vi "Disconnect SMU Resources from site.vi"(0 "TSM context":T1, 5 "Site Relays(T)/Non-Site(F)?":bool, 11 "error in":errorcluster) -> (4 "TSM context out":T1, 15 "error out":errorcluster)   [LabVIEW 2019]
doc: "This VI is used to disconnect SMU resources safely by preventing potetial OCP errors."
uses:
  <vilib>/NI_TestStand_SemiconductorModule/NI_TestStand_Semiconductor_Module.lvlibp/PinMap/General/SemiconductorModuleContext.ctl
  <vilib>/NI_TestStand_SemiconductorModule/NI_TestStand_Semiconductor_Module.lvlibp/PinMap/General/NIInstrumentTypeIDs.ctl
  <instrlib>/niDCPower/nidcpower.llb/niDCPower Output Function.ctl
  <instrlib>/niDCPower/nidcpower.llb/niDCPower Sense.ctl
  <instrlib>/niDCPower/nidcpower.llb/niDCPower Source Mode.ctl
  TSM Context Data Access/Public/Properties/TestFlowID - Read.vi
  <vilib>/NI_TestStand_SemiconductorModule/NI_TestStand_Semiconductor_Module.lvlibp
  TSM Context Data Access/TSM Context Data Access.lvclass
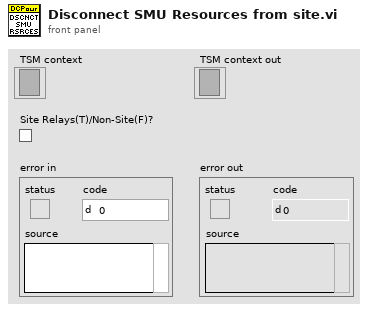
[diagram p1: front panel]
types:
  T1 = typedef "NI_TestStand_Semiconductor_Module.lvlibp/SemiconductorModuleContext.ctl" = refnum<k7>
  T2 = typedef "niDCPower Source Mode.ctl" = i32
  T3 = typedef "niDCPower Sense.ctl" = i32
  T4 = typedef "niDCPower Output Function.ctl" = i32
  T5 = typedef "NI_TestStand_Semiconductor_Module.lvlibp/NIInstrumentTypeIDs.ctl" = string
  T6 = typedef "TSM SSC DCPower.ctl" = cluster{"Pin Query Context":refnum<class "MultiplePinMultipleSessionQueryContext.lvclass">, "SSC":T7[], "Site Numbers":i32[], "Pins":T8[], "Pins Expanded":T10[]}
  T7 = typedef "SSC DCPower.ctl" = cluster{"Session":refnum<k15>, "Chan":string, "Channel List":string}
  T8 = typedef "TSM Pin Information.ctl" = cluster{"Pin":tag, "Type":T9, "Count":i32}
  T9 = typedef "TSM Pin Type Identifier.ctl" = enum8{"DUT Pin", "System Pin", "Pin Group", "Not Determined"}
  T10 = typedef "TSM Expanded Pin Information.ctl" = cluster{"Pin":tag, "Type":T9, "Index":i32}
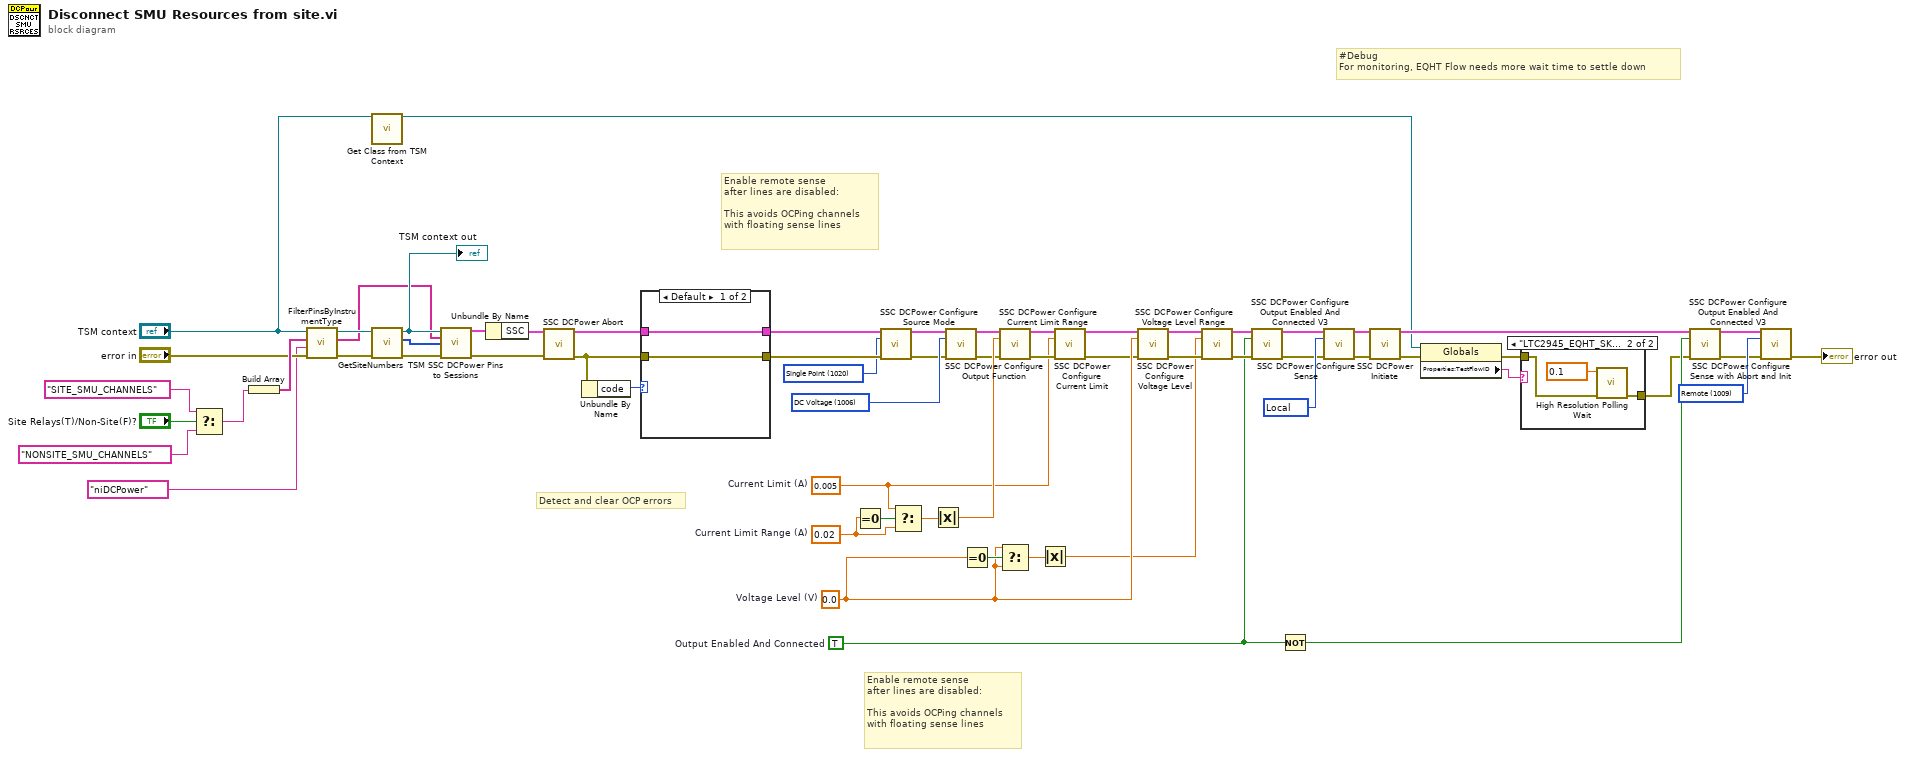
[diagram p0: block diagram]
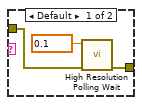
[diagram p2: hidden frame]
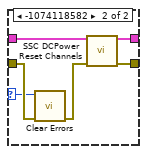
[diagram p3: hidden frame]
diagram:
  w16 = T2 1020 items=["Single Point"=1020, "Sequence"=1021] ("Source Mode")
  w21 = T3 1009 items=["Local"=1008, "Remote"=1009] ("Sense")
  w29 = T3 1008 items=["Local"=1008, "Remote"=1009] ("Sense")
  w42 = T4 1006 items=["DC Voltage"=1006, "DC Current"=1007, "Pulse Voltage"=1049, "Pulse Current"=1050] ("Output Function")
  w41 = 0.005  # Current Limit (A)
  w39 = 0.0  # Voltage Level (V)
  w40 = 0.02  # Current Limit Range (A)
  w13 = TRUE  # Output Enabled And Connected
  # "#Debug\nFor monitoring, EQHT Flow needs more wait time to settle down"
  # "Enable remote sense\nafter lines are disabled:\n\nThis avoids OCPing channels\nwith floating sense lines"
  # "Enable remote sense\nafter lines are disabled:\n\nThis avoids OCPing channels\nwith floating sense lines"
  # "Detect and clear OCP errors"
  n1 = Select(t="SITE_SMU_CHANNELS", s="Site Relays(T)/Non-Site(F)?", f="NONSITE_SMU_CHANNELS") -> (s? t:f=w25:string)
  n2 = Build Array(w25) -> (w52:string[])
  n3 = call <vilib>:"FilterPinsByInstrumentType.vi"("error in (no error)"="error in", "Instrument Type Id"=T5 "niDCPower", "Pins"=w52, "Semiconductor Module Context"="TSM context") -> ("error out"=w59:errorcluster, "Filtered Pins"=w53:tag[], "Semiconductor Module Context Out"=w56:T1)  [unwired: 5 in]
  n4 = call "Get Class from TSM Context.vi"("TSM Context"="TSM context") -> ("Global Memory Class"=w3:refnum<class "TSM Context Data Access.lvclass">)  [unwired: 14 in]
  n5 = call <vilib>:"GetSiteNumbers.vi"("error in (no error)"=w59, "Semiconductor Module Context"=w56) -> ("error out"=w57:errorcluster, "Site Numbers"=w54:i32[], "Semiconductor Module Context Out"=w55:T1)  [unwired: 6 in, 1 out]
  "TSM context out" <- w55
  n6 = call "TSM SSC DCPower Pins to Sessions.vi"("TSM context"=w55, "Pins"=w53, "Site Numbers"=w54, "error in"=w57) -> ("DCPower TSM Out"=w60:T6, "error out"=w38:errorcluster)  [unwired: 10 in]
  n7 = Unbundle By Name(w60) -> ("SSC"=w37:T7[])
  n8 = call "SSC DCPower Abort.vi"("DCPower SSC in"=w37, "error in"=w38) -> ("DCPower SSC out"=w58:T7[], "error out"=w61:errorcluster)  [unwired: 12 in]
  n9 = Unbundle By Name(w61) -> ("code"=w62:i32)
  n10 = case shown="Default" w62 {
    selector: w62 -> [_ w67]
    tunnel: [w64 w69] -> w20
    tunnel: w61 -> [w64 w70]
    tunnel: w58 -> [w63 w66]
    tunnel: [w63 w65] -> w19
    frame Default {
    }
    frame -1074118582 {
      n11 = call <vilib>:"Clear Errors.vi"("error in (no error)"=w70, "specific error code to clear (0: all)"=w67) -> ("error out"=w68:errorcluster)  [unwired: 4 in, 1 out]
      n12 = call "SSC DCPower Reset Channels.vi"("DCPower SSC in"=w66, "error in"=w68) -> ("DCPower SSC out"=w65:T7[], "error out"=w69:errorcluster)  [unwired: 12 in]
    }
  }
  n13 = Equal To 0?(x=w40) -> (x = 0?=w50:bool)
  n14 = call "SSC DCPower Configure Source Mode.vi"("DCPower SSC in"=w19, "Source Mode"=w16, "error in"=w20) -> ("DCPower SSC out"=w17:T7[], "error out"=w18:errorcluster)  [unwired: 11 in]
  n15 = Select(t=w41, s=w50, f=w40) -> (s? t:f=w49:dbl)
  n16 = Absolute Value(x=w49) -> (abs(x)=w51:dbl)
  n17 = call "SSC DCPower Configure Output Function.vi"("DCPower SSC in"=w17, "Output Function"=w42, "error in"=w18) -> ("DCPower SSC out"=w43:T7[], "error out"=w44:errorcluster)  [unwired: 11 in]
  n18 = Equal To 0?(x=w39) -> (x = 0?=w47:bool)
  n19 = call "SSC DCPower Configure Current Limit Range.vi"("DCPower SSC in"=w43, "Current Limit Range (A)"=w51, "error in"=w44) -> ("DCPower SSC out"=w45:T7[], "error out"=w46:errorcluster)  [unwired: 11 in]
  n20 = Select(t=w39, s=w47, f=w39) -> (s? t:f=w48:dbl)
  n21 = Absolute Value(x=w48) -> (abs(x)=w32:dbl)
  n22 = call "SSC DCPower Configure Current Limit.vi"("DCPower SSC in"=w45, "Current Limit (A)"=w41, "error in"=w46) -> ("DCPower SSC out"=w35:T7[], "error out"=w36:errorcluster)  [unwired: 11 in]
  n23 = call "SSC DCPower Configure Voltage Level.vi"("DCPower SSC in"=w35, "Voltage Level (V)"=w39, "error in"=w36) -> ("DCPower SSC out"=w33:T7[], "error out"=w34:errorcluster)  [unwired: 11 in]
  n24 = call "SSC DCPower Configure Voltage Level Range.vi"("DCPower SSC in"=w33, "Voltage Level Range (V)"=w32, "error in"=w34) -> ("DCPower SSC out"=w14:T7[], "error out"=w15:errorcluster)  [unwired: 11 in]
  n25 = call "SSC DCPower Configure Output Enabled And Connected V3.vi"("DCPower SSC in"=w14, "Output Enabled And Connected"=w13, "error in"=w15) -> ("DCPower SSC out"=w11:T7[], "error out"=w12:errorcluster)  [unwired: 11 in]
  n26 = Not(x=w13) -> (.not. x?=w7:bool)
  n27 = call "SSC DCPower Configure Sense.vi"("DCPower SSC in"=w11, "Sense"=w29, "error in"=w12) -> ("DCPower SSC out"=w27:T7[], "error out"=w28:errorcluster)  [unwired: 11 in]
  n28 = call "SSC DCPower Initiate.vi"("DCPower SSC in"=w27, "error in"=w28) -> ("DCPower SSC out"=w9:T7[], "error out"=w4:errorcluster)  [unwired: 12 in]
  n29 = property class="Globals"(reference=w3, error in=w4) -> (error out=w2:errorcluster, "Properties:TestFlowID"=w1:string)  [unwired: 1 out]
  n30 = case shown="\"LTC2945_EQHT_SKIP_TRIM\"" w1 {
    tunnel: [w72 w75] -> w6
    tunnel: w2 -> [w71 w74]
    frame Default {
      n31 = call <vilib>:"High Resolution Polling Wait.vi"("error in (no error)"=w71, "seconds to wait"=0.1) -> ("error out"=w72:errorcluster)  [unwired: 9 in]
    }
    frame "LTC2945_EQHT_SKIP_TRIM" {
      n32 = call <vilib>:"High Resolution Polling Wait.vi"("error in (no error)"=w74, "seconds to wait"=0.1) -> ("error out"=w75:errorcluster)  [unwired: 9 in]
    }
  }
  n33 = call "SSC DCPower Configure Output Enabled And Connected V3.vi"("DCPower SSC in"=w9, "Output Enabled And Connected"=w7, "error in"=w6) -> ("DCPower SSC out"=w8:T7[], "error out"=w10:errorcluster)  [unwired: 11 in]
  n34 = call "SSC DCPower Configure Sense with Abort and Init.vi"("DCPower SSC in"=w8, "Sense"=w21, "error in"=w10) -> ("error out"=→"error out":errorcluster)  [unwired: 11 in, 1 out]
